vi "New Default Lookup.vi"(8 "error in (no error)":errorcluster) -> (0 "error out":errorcluster, 3 "New Default Lookup":refnum<data-value>)   [LabVIEW 2019, in "Default Lookup.lvclass"]
doc: "Create new Default Lookup instance. A Lookup is a map of object instances to a specific base class."
uses:
  Default Lookup.lvclass
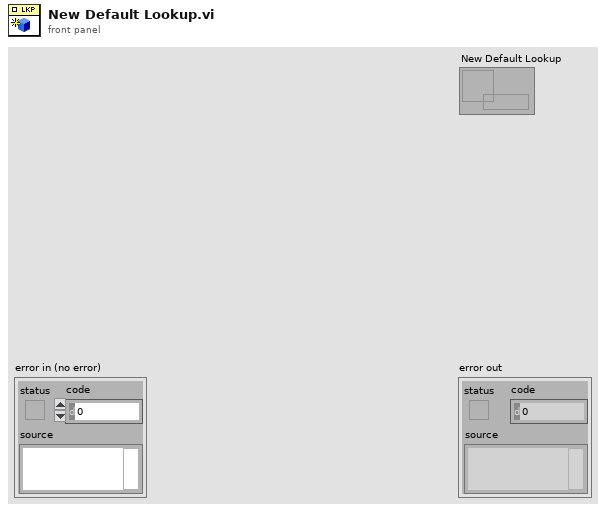
[diagram p1: front panel]
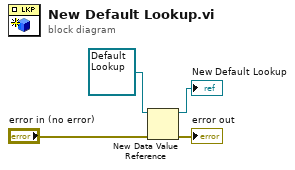
[diagram p0: block diagram]
diagram:
  n1 = New Data Value Reference(data value=refnum<class "Default Lookup.lvclass"> refnum ("Default Lookup in"), error in="error in (no error)") -> (data value reference=→"New Default Lookup":refnum<data-value>, error out=→"error out":errorcluster)
